vi "Wavegen_SimpleConfig.vi"(8 "error in (no error)":errorcluster caption="错误输入（无错误）", 9 "CalArray":u8[](array[numeric]), 10 "参数":T1={"ch"=1, "amp"=1.0, "vOffset"=0.0, "hzFrequency"=2000, "percentageSymmetry"=50.0, "degreePhase"=0.0, "func"=enum."Sine"}, 11 "ftHandle":u64) -> (0 "error out":errorcluster caption="错误输出", 2 "function out":i32, 3 "ftHandle out":u64)   [LabVIEW 2018]
doc: "Set Wavegen Simple mode configration .\nch:0,1\nfunc:0-10 dc,sine...\namp:0-5V\noffset:-5~5V\nsymmetry:0~100 %\nphase:0~360 °\nfrequency:1~20MHz"
uses:
  InstrumentsPlayground.lvlib
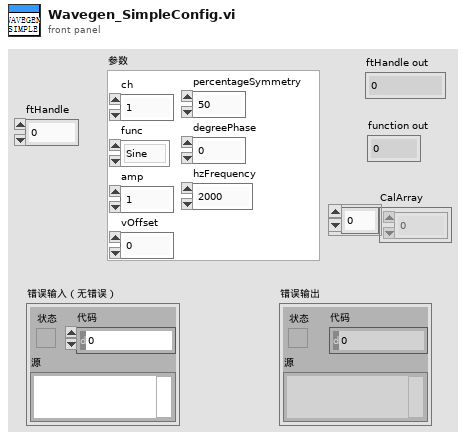
[diagram p1: front panel]
types:
  T1 = cluster{"ch":i32, "amp":dbl, "vOffset":dbl, "hzFrequency":i32, "percentageSymmetry":dbl, "degreePhase":dbl, "func":enum8{"DC", "Sine", "Square", "Triangle", "RampUp", "RampDown", "Noise", "Pulse", "Trapezium", "SinePower", "Custom", "Play"}}
  T2 = enum8{"DC", "Sine", "Square", "Triangle", "RampUp", "RampDown", "Noise", "Pulse", "Trapezium", "SinePower", "Custom", "Play"}
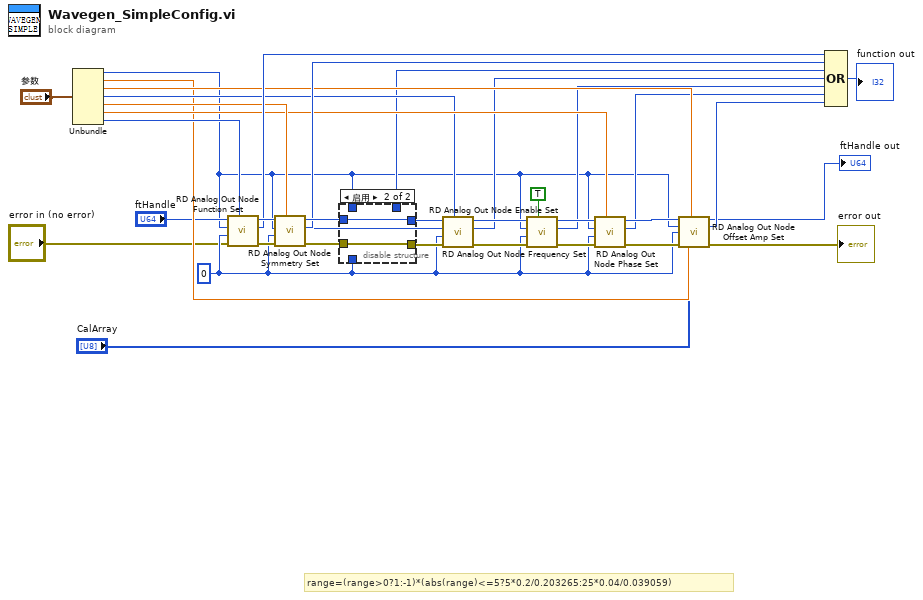
[diagram p0: block diagram]
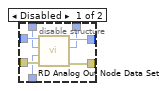
[diagram p2: hidden frame]
diagram:
  w23 = 0 ("node")
  # "range=(range>0?1:-1)*(abs(range)<=5?5*0.2/0.203265:25*0.04/0.039059)"
  n1 = Unbundle("参数") -> ("ch"=w2:i32, "amp"=w13:dbl, "vOffset"=w14:dbl, "hzFrequency"=w15:i32, "percentageSymmetry"=w17:dbl, "degreePhase"=w16:dbl, "func"=w18:T2)
  n2 = call "RD Analog Out Node Function Set.vi"("func"=w18, "error in (no error)"="error in (no error)", "node"=w23, "ch"=w2, "handle"="ftHandle") -> ("error out"=w26:errorcluster, "function return"=w22:i32, "handle out"=w27:u64)  [unwired: 4 in]
  n3 = call "RD Analog Out Node Symmetry Set.vi"("percentageSymmetry"=w17, "error in (no error)"=w26, "node"=w23, "ch"=w2, "handle"=w27) -> ("error out"=w31:errorcluster, "function return"=w21:i32, "handle out"=w35:u64)  [unwired: 4 in]
  n4 = disable-structure shown="启用" {
    disable-tunnel: w35 -> [w42 w44]
    disable-tunnel: [w41 w44] -> w34
    disable-tunnel: w31 -> [w40 w43]
    disable-tunnel: [w39 w43] -> w30
    disable-tunnel: w23 -> [w38 _]
    disable-tunnel: w2 -> [w37 _]
    disable-tunnel: [w36 _] -> w10
    frame Disabled {
      n5 = call "RD Analog Out Node Data Set.vi"("error in (no error)"=w40, "node"=w38, "ch"=w37, "handle"=w42) -> ("error out"=w39:errorcluster, "function return"=w36:i32, "handle out"=w41:u64)  [unwired: 4 in, 1 out]
    }
    frame Enabled {
    }
  }
  n6 = call "RD Analog Out Node Frequency Set.vi"("hzFrequency"=w15, "error in (no error)"=w30, "node"=w23, "ch"=w2, "handle"=w34) -> ("error out"=w29:errorcluster, "function return"=w9:i32, "handle out"=w33:u64)  [unwired: 4 in]
  n7 = call "RD Analog Out Node Enable Set.vi"("enable"=TRUE, "error in (no error)"=w29, "node"=w23, "ch"=w2, "handle"=w33) -> ("error out"=w25:errorcluster, "function return"=w8:i32, "handle out"=w24:u64)  [unwired: 4 in]
  n8 = call "RD Analog Out Node Phase Set.vi"("degreePhase"=w16, "error in (no error)"=w25, "node"=w23, "ch"=w2, "handle"=w24) -> ("error out"=w28:errorcluster, "function return"=w7:i32, "handle out"=w32:u64)  [unwired: 4 in]
  n9 = call "RD Analog Out Node Offset Amp Set.vi"("handle"=w32, "amp"=w13, "ch"=w2, "node"=w23, "vOffset"=w14, "error in (no error)"=w28, "CalArray"="CalArray") -> ("handle out"=→"ftHandle out":u64, "function return"=w6:i32, "error out"=→"error out":errorcluster)  [unwired: 5 in, 1 out]
  n10 = Compound Arithmetic op=OR ("复合运算")(w22, w21, w10, w9, w8, w7, w6) -> (→"function out":i32)
